vi "read_attributes.vi"(8 "error in (no error)":errorcluster, 11 "Birch in":refnum<class "Birch.lvclass">) -> (0 "error out":errorcluster, 2 "attributes":T1, 3 "Birch out":refnum<class "Birch.lvclass">)   [LabVIEW 2020, in "Birch.lvclass"]
uses:
  Birch.lvclass
  Controls/birch_attributes.ctl
  Birch.lvclass/Birch.ctl
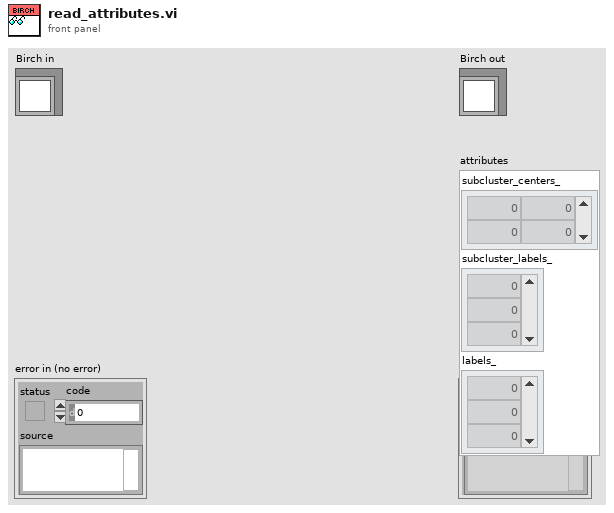
[diagram p1: front panel]
types:
  T1 = typedef "birch_attributes.ctl" = cluster{"subcluster_centers_":dbl[][], "subcluster_labels_":dbl[], "labels_":dbl[]}
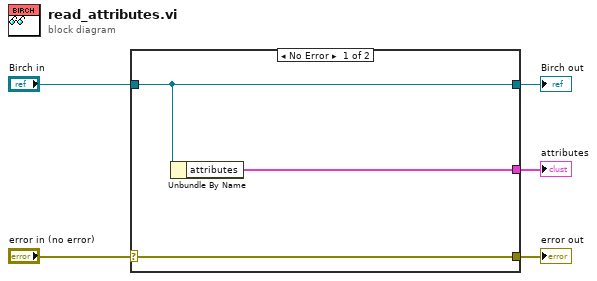
[diagram p0: block diagram]
diagram:
  n1 = case shown="No Error" "error in (no error)" {
    selector: "error in (no error)" -> [w8 w9]
    tunnel: [w8 w9] -> w4
    tunnel: [w7 w10] -> w2
    tunnel: "Birch in" -> [w7 w10]
    tunnel: [w6 _] -> w1
    frame No Error {
      n2 = Unbundle By Name(w7) -> ("attributes"=w6:T1)
    }
    frame Error {
    }
  }
  "error out" <- w4
  "Birch out" <- w2
  "attributes" <- w1
